vi "Decompose LabVIEW Object - String - Private Data Cluster Count.vi"() -> ()   [LabVIEW 2017, in "Composition.Tests.lvlib"]
uses:
  Composition.Tests.lvlib
  Classes/String/String.lvclass
  Composition/Composition.lvlib
  <vilib>/addons/_JKI Toolkits/Caraya/classes/Assert/Assert.lvclass
  <vilib>/addons/_JKI Toolkits/Caraya/classes/Test/Test.lvclass
panel:
  out "error out":errorcluster
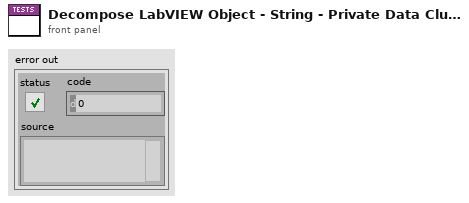
[diagram p1: front panel]
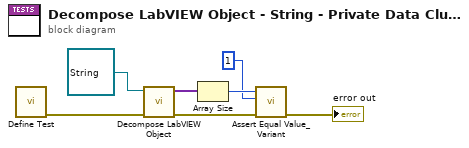
[diagram p0: block diagram]
diagram:
  n1 = call <vilib>:"Define Test.vi"() -> ("error out"=w1:errorcluster)  [unwired: 11 in]
  n2 = call "Decompose LabVIEW Object.vi"("error in (no error)"=w1, "LabVIEW Object"=refnum<class "String.lvclass"> refnum ("Reflection.Tests.lvlib:String.lvclass")) -> ("error out"=w6:errorcluster, "Private Data Clusters"=w4:variant[])  [unwired: 6 in, 2 out]
  n3 = Array Size(array=w4) -> (size(s)=w3:i32)
  n4 = call <vilib>:"Assert Equal Value_Variant.vi"("error in (no error)"=w6, "Y"=1 ("Expected"), "X"=w3) -> ("error out"=→"error out":errorcluster)  [unwired: 8 in]
